vi "Вычислительное_устройство.vi"(0 "Minus":bool, 1 "Keyboard":T4, 2 "Reset":bool, 3 "Cinp":bool, 4 "c":bool, 5 "selInp":bool, 6 "selOp":bool, 7 "Cread":bool, 8 "Adr A":cluster{"a0":bool, "a1":bool}, 9 "Adr b":cluster{"a0":bool, "a1":bool}, 10 "wr":bool, 11 "Exec":bool, 12 "ClearAcc":bool, 13 "Func":T1, 14 "read":bool) -> (20 "sign":bool, 21 "dig0":T2, 22 "dig1":T2, 23 "flags":T3)   [LabVIEW 2013]
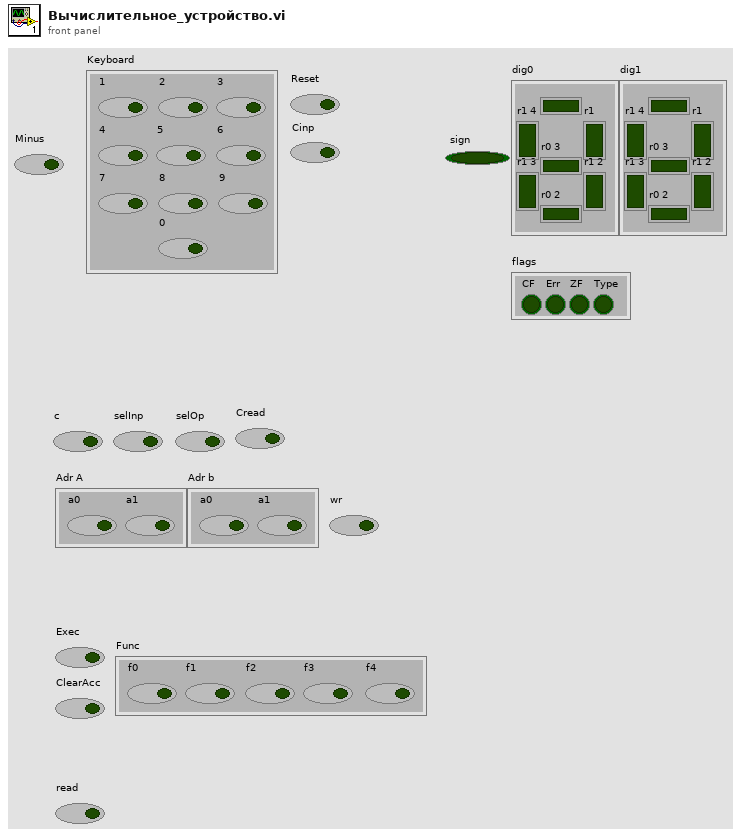
[diagram p1: front panel]
types:
  T1 = cluster{"f0":bool, "f1":bool, "f2":bool, "f3":bool, "f4":bool}
  T2 = cluster{"r0":bool, "r1":bool, "r1 2":bool, "r0 2":bool, "r1 3":bool, "r1 4":bool, "r0 3":bool}
  T3 = cluster{"CF":bool, "Err":bool, "ZF":bool, "Type":bool}
  T4 = cluster{"0":bool, "1":bool, "2":bool, "3":bool, "4":bool, "5":bool, "6":bool, "7":bool, "8":bool, "9":bool}
  T5 = cluster{"n0":bool, "n1":bool, "n2":bool, "n3":bool, "n4":bool}
  T6 = cluster{"r0":bool, "r1":bool, "r2":bool, "r3":bool, "r4":bool}
  T7 = cluster{"r0":bool, "r1":bool, "r2":bool, "r3":bool}
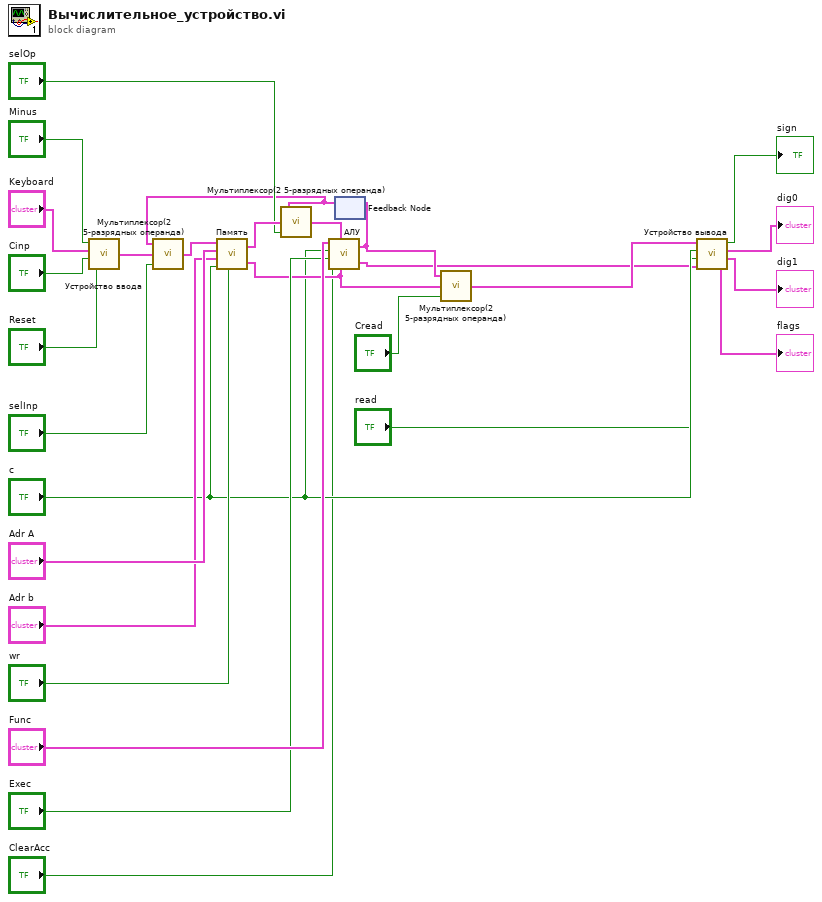
[diagram p0: block diagram]
diagram:
  n1 = call "Устройство ввода.vi"("Reset"="Reset", "c"="Cinp", "Keyboard"="Keyboard", "Minus"="Minus") -> ("N"=w19:T5)
  n2 = feedback #1() -> (w9:T6)  [unwired: 1 in]
  n3 = call "Мультиплексор(2 5-разрядных операнда).vi"("c"="selInp", "Inp1"=w19, "Inp0"=w9) -> ("r"=w18:T6)
  n4 = call "Память.vi"("Inp"=w18, "Adr A"="Adr A", "Adr b"="Adr b", "c"="c", "wr"="wr") -> ("A"=w11:T6, "B"=w8:T6)
  n5 = call "Мультиплексор(2 5-разрядных операнда).vi"("c"="selOp", "Inp1"=w11, "Inp0"=w9) -> ("r"=w12:T6)
  n6 = call "АЛУ.vi"("B"=w8, "A"=w12, "ClearAcc"="ClearAcc", "Exec"="Exec", "c"="c", "Func"="Func") -> ("Flags"=w2:T3, "R"=w7:T6)
  n7 = feedback-in #1(w7) -> ()
  n8 = call "Мультиплексор(2 5-разрядных операнда).vi"("c"="Cread", "Inp1"=w8, "Inp0"=w7) -> ("r"=w5:T6)
  n9 = call "Устройство вывода.vi"("F"=w2, "read"="read", "c"="c", "A"=w5) -> ("flags"=→"flags":T7, "dig1"=→"dig1":T2, "dig0"=→"dig0":T2, "sign"=→"sign":bool)
